vi "switches_to_number.vi"(4 "error in (no error)":errorcluster, 7 "switches":bool[](array[boolean])=[FALSE, FALSE, FALSE, FALSE, FALSE, FALSE, FALSE, FALSE]) -> (0 "error out":errorcluster, 3 "number":u8)   [LabVIEW 2018]
doc: "convertes a bollean array with 8 switches to a number. This is used to convert the status of the switches to the a number (the \"data\") that can be send to the controller"
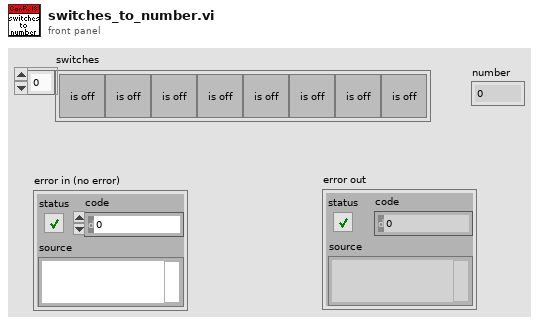
[diagram p1: front panel]
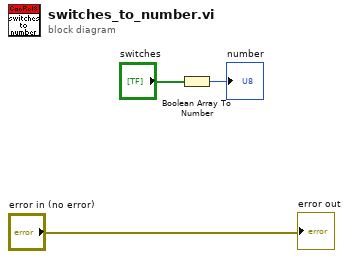
[diagram p0: block diagram]
diagram:
  n1 = Boolean Array To Number(Boolean array="switches") -> (number=→"number":u32)
  "error out" <- "error in (no error)"
